vi "Read.vi"(8 "Error In":errorcluster, 11 "Xbox One Controller Ref":T3) -> (0 "Error Out":errorcluster, 1 "All Axis":T1, 2 "Buttons":T4, 3 "Xbox One Controller Ref":T3)   [LabVIEW 2011, in "LVH-Xbox-One-Controller.lvlib"]
uses:
  LVH-Xbox-One-Controller.lvlib
  Private/Type Defs/Xbox One Controller Ref.ctl
  Private/Type Defs/Indicators/All Buttons Visual.ctl
  Private/Type Defs/Indicators/A.ctl
  Private/Type Defs/Indicators/B.ctl
  Private/Type Defs/Indicators/X.ctl
  Private/Type Defs/Indicators/Y.ctl
  Private/Type Defs/Indicators/Left Bumper.ctl
  Private/Type Defs/Indicators/Right Bumper.ctl
  Private/Type Defs/Indicators/View.ctl
  Private/Type Defs/Indicators/Menu.ctl
  Private/Type Defs/Indicators/Thumbstick.ctl
  Private/Type Defs/Indicators/All Axis Data.ctl
  Private/Type Defs/Indicators/DPad Enum.ctl
  <vilib>/Utility/inputDevices.llb/joystickAcquire.vi
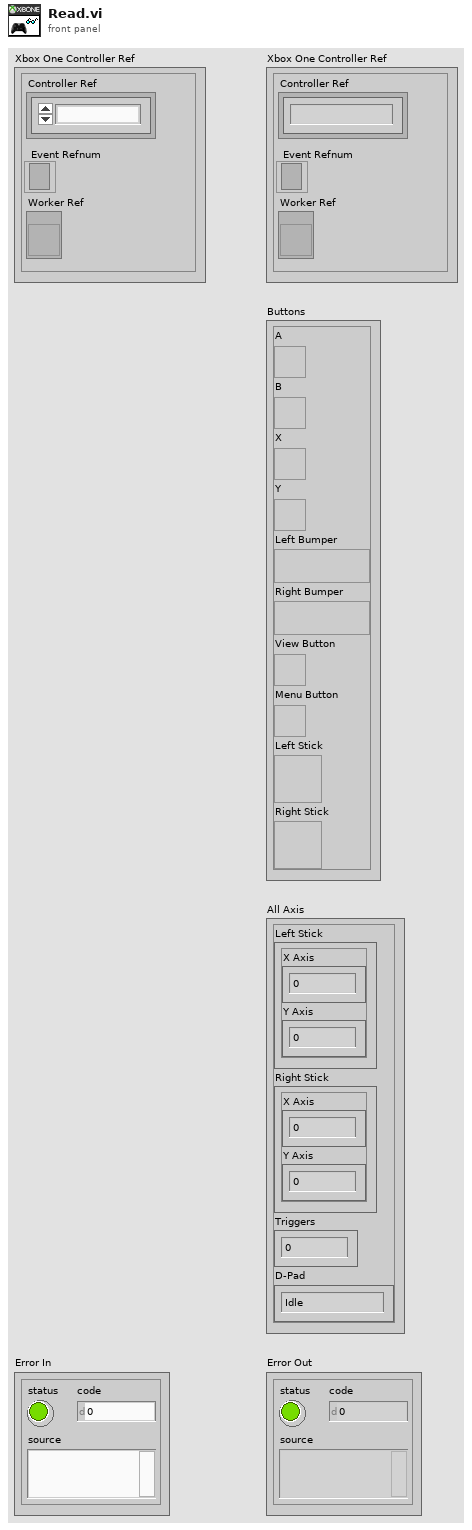
[diagram p1: front panel]
types:
  T1 = typedef "LVH-Xbox-One-Controller.lvlib/All Axis Data.ctl" = cluster{"Left Stick":cluster{"X Axis":i32, "Y Axis":i32}, "Right Stick":cluster{"X Axis":i32, "Y Axis":i32}, "Triggers":i32, "D-Pad":T2}
  T2 = typedef "LVH-Xbox-One-Controller.lvlib/DPad Enum.ctl" = enum16{"Idle", "Up", "Up / Right", "Right", "Down / Right", "Down", "Down / Left", "Left", "Up / Left"}
  T3 = typedef "LVH-Xbox-One-Controller.lvlib/Xbox One Controller Ref.ctl" = cluster{"Controller Ref":refnum<k1>, "Event Refnum":refnum<event-registration>, "Worker Ref":refnum<vi>}
  T4 = typedef "LVH-Xbox-One-Controller.lvlib/All Buttons Visual.ctl" = cluster{"A":T5, "B":T6, "X":T7, "Y":T8, "Left Bumper":T9, "Right Bumper":T10, "View Button":T11, "Menu Button":T12, "Left Stick":T13, "Right Stick":T13}
  T5 = typedef "LVH-Xbox-One-Controller.lvlib/A.ctl" = bool
  T6 = typedef "LVH-Xbox-One-Controller.lvlib/B.ctl" = bool
  T7 = typedef "LVH-Xbox-One-Controller.lvlib/X.ctl" = bool
  T8 = typedef "LVH-Xbox-One-Controller.lvlib/Y.ctl" = bool
  T9 = typedef "LVH-Xbox-One-Controller.lvlib/Left Bumper.ctl" = bool
  T10 = typedef "LVH-Xbox-One-Controller.lvlib/Right Bumper.ctl" = bool
  T11 = typedef "LVH-Xbox-One-Controller.lvlib/View.ctl" = bool
  T12 = typedef "LVH-Xbox-One-Controller.lvlib/Menu.ctl" = bool
  T13 = typedef "LVH-Xbox-One-Controller.lvlib/Thumbstick.ctl" = bool
  T14 = cluster{"X axis":i32, "Y axis":i32, "Z axis":i32, "X axis rotation":i32, "Y axis rotation":i32, "Z axis rotation":i32, "U axis":i32, "V axis":i32}
  T15 = cluster{"button 1":bool, "button 2":bool, "button 3":bool, "button 4":bool, "button 5":bool, "button 6":bool, "button 7":bool, "button 8":bool, "button 9":bool, "button 10":bool, "button 11":bool, "button 12":bool, "button 13":bool, "button 14":bool, "button 15":bool, "button 16":bool, "button 17":bool, "button 18":bool, "button 19":bool, "button 20":bool, "button 21":bool, "button 22":bool, "button 23":bool, "button 24":bool, "button 25":bool, "button 26":bool, "button 27":bool, "button 28":bool, "button 29":bool, "button 30":bool, "button 31":bool, "button 32":bool}
  T16 = cluster{"pov 1":i32, "pov 2":i32, "pov 3":i32, "pov 4":i32}
  T17 = cluster{"X axis rotation":i32, "Y axis rotation":i32}
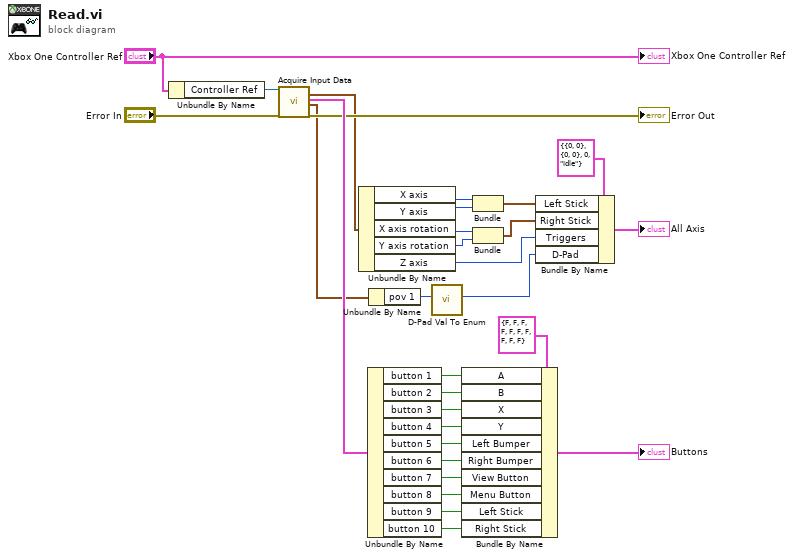
[diagram p0: block diagram]
diagram:
  n1 = Unbundle By Name("Xbox One Controller Ref") -> ("Controller Ref"=w29:refnum<k1>)
  n2 = call-poly <vilib>:"Acquire Input Data.vi"("device ID"=w29, "error in (no error)"="Error In") -> ("axis info"=w13:T14, "button info"=w26:T15, "direction info"=w4:T16, "error out"=→"Error Out":errorcluster)  [unwired: 13 in, 1 out]
  n3 = Unbundle By Name(w13) -> ("X axis"=w10:i32, "Y axis"=w11:i32, "X axis rotation"=w9:i32, "Y axis rotation"=w8:i32, "Z axis"=w5:i32)
  n4 = Unbundle By Name(w26) -> ("button 1"=w24:bool, "button 2"=w23:bool, "button 3"=w22:bool, "button 4"=w21:bool, "button 5"=w20:bool, "button 6"=w19:bool, "button 7"=w18:bool, "button 8"=w17:bool, "button 9"=w16:bool, "button 10"=w15:bool)
  n5 = Unbundle By Name(w4) -> ("pov 1"=w3:i32)
  n6 = call "D-Pad Val To Enum.vi"("D-Pad Value"=w3) -> ("D-Pad Enum"=w2:T2)  [unwired: 10 in]
  n7 = Bundle By Name(cluster=T4 {"A"=FALSE, "B"=FALSE, "X"=FALSE, "Y"=FALSE, "Left Bumper"=FALSE, "Right Bumper"=FALSE, "View Button"=FALSE, "Menu Button"=FALSE, "Left Stick"=FALSE, "Right Stick"=FALSE} ("Buttons"), "A"=w24, "B"=w23, "X"=w22, "Y"=w21, "Left Bumper"=w20, "Right Bumper"=w19, "View Button"=w18, "Menu Button"=w17, "Left Stick"=w16, "Right Stick"=w15) -> (→"Buttons":T4)
  n8 = Bundle("X axis"=w10, "Y axis"=w11) -> (w7:cluster{"X axis":i32, "Y axis":i32})  [unwired: 1 in]
  n9 = Bundle("X axis rotation"=w9, "Y axis rotation"=w8) -> (w6:T17)  [unwired: 1 in]
  n10 = Bundle By Name(cluster=T1 {"Left Stick"={"X Axis"=0, "Y Axis"=0}, "Right Stick"={"X Axis"=0, "Y Axis"=0}, "Triggers"=0, "D-Pad"=enum."Idle"} ("All Axis Data"), "Left Stick"=w7, "Right Stick"=w6, "Triggers"=w5, "D-Pad"=w2) -> (→"All Axis":T1)
  "Xbox One Controller Ref" <- "Xbox One Controller Ref"
